vi "Control Valve.vi"(0 "Session Handle in":T2, 5 "Valves":T1=52 items=["GV1"=21, ""=0], 7 "Energize?":bool, 11 "error in (no error)":errorcluster) -> (4 "Session Handle out":T2, 6 "Success?":bool, 15 "error out":errorcluster)   [LabVIEW 2015, in "Gas.lvclass"]
uses:
  Gas.lvclass
  Typedefs/Session Handle.ctl
  Typedefs/Valves.ctl
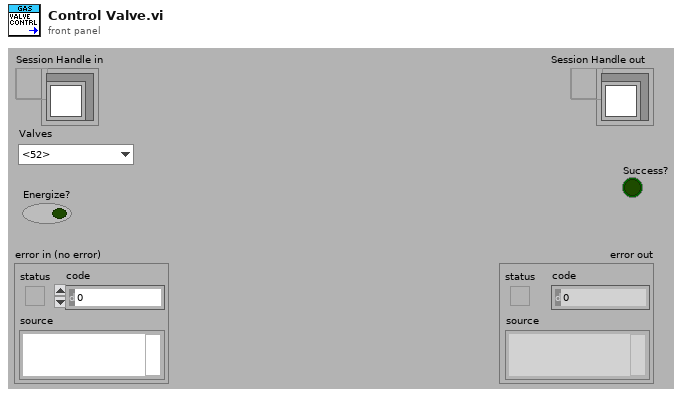
[diagram p1: front panel]
types:
  T1 = typedef "Gas.lvclass/Valves.ctl" = u16
  T2 = typedef "Gas.lvclass/Session Handle.ctl" = refnum<data-value>
  T3 = typedef "XNET Frame CAN.ctl" = cluster{"timestamp":timestamp, "payload":u8[], "identifier":u32, "type":T4, "extended?":bool, "echo?":bool}
  T4 = typedef "XNET Frame Type CAN.ctl" = u8
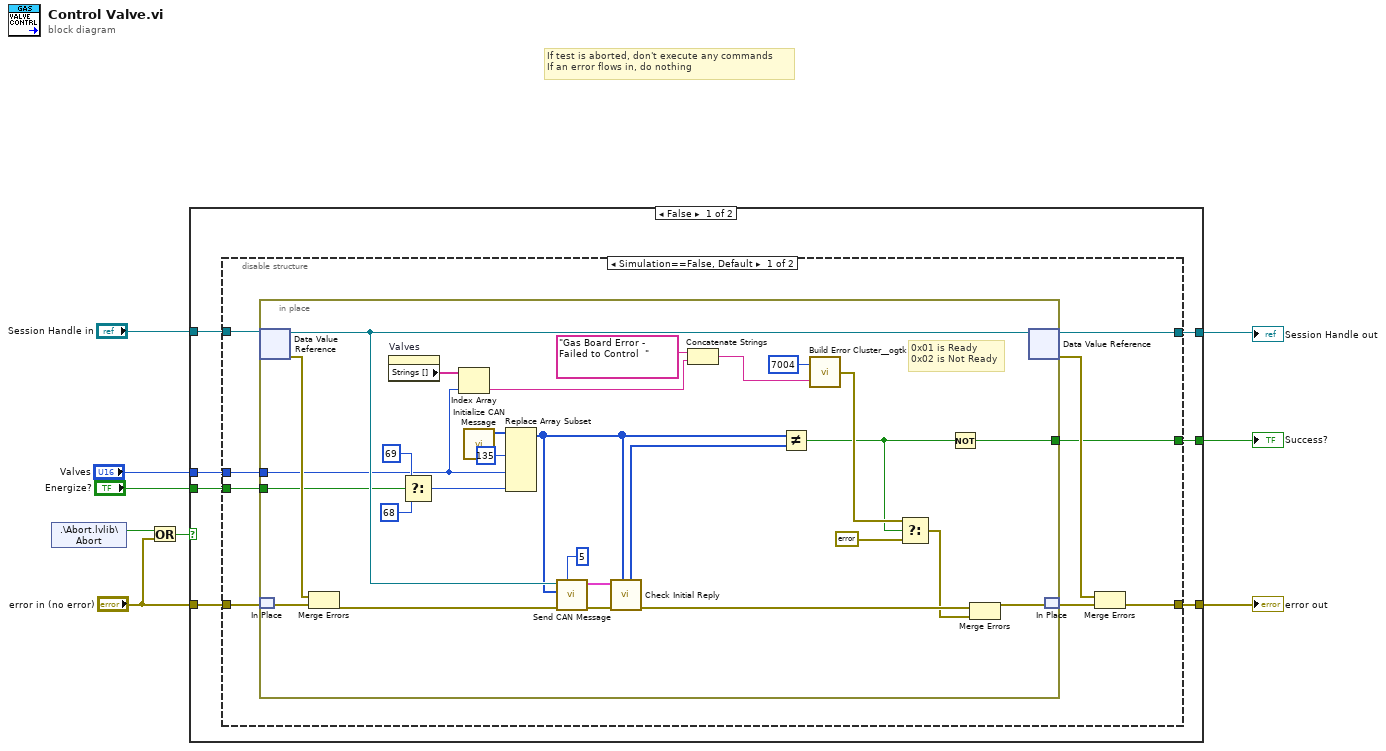
[diagram p0: block diagram]
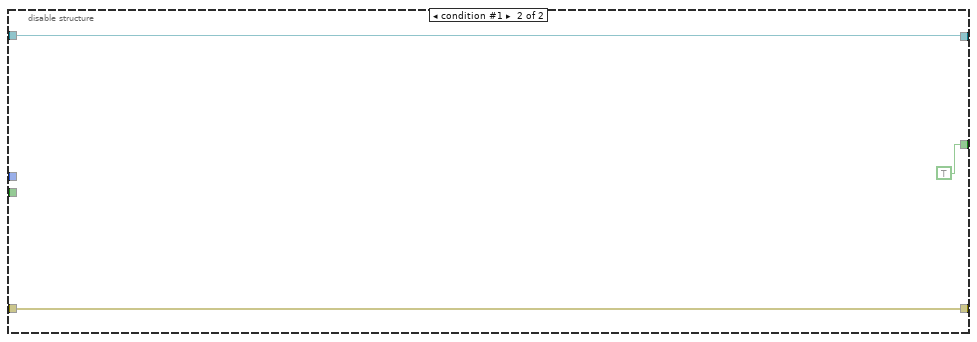
[diagram p2: hidden frame]
diagram:
  # "If test is aborted, don't execute any commands\nIf an error flows in, do nothing"
  n1 = shared-variable ".\\Abort.lvlib\\Abort"() -> (w6:bool)  [unwired: 1 in, 1 out]
  n2 = Or(x=w6, y="error in (no error)") -> (x .or. y?=w4:bool)
  n3 = case shown="False" w4 {
    tunnel: [w16 w58] -> w8
    tunnel: [w15 w57] -> w7
    tunnel: "Session Handle in" -> [w14 w58]
    tunnel: "error in (no error)" -> [w13 w57]
    tunnel: [w12 _] -> w3
    tunnel: "Valves" -> [w11 _]
    tunnel: "Energize?" -> [w10 _]
    frame False {
      n4 = disable-structure shown="Simulation==False, Default" {
        disable-tunnel: [w25 w56] -> w16
        disable-tunnel: [w22 w55] -> w15
        disable-tunnel: w14 -> [w21 w56]
        disable-tunnel: w13 -> [w20 w55]
        disable-tunnel: [w19 TRUE] -> w12
        disable-tunnel: w11 -> [w18 _]
        disable-tunnel: w10 -> [w17 _]
        frame condition #0 (active) {
          n5 = in-place {
            in-place-border: [w40] -> w19
            in-place-border: w18 -> [w32]
            in-place-border: w17 -> [w39]
            # "0x01 is Ready\n0x02 is Not Ready"
            n6 = in-place-dvr #1(w21) -> (w47:refnum<class "Gas.lvclass">, w50:errorcluster)
            n7 = in-place-match #2(w20) -> (w49:errorcluster)
            n8 = Merge Errors(w50, w49) -> (w48:errorcluster)
            n9 = property on="Valves" class="Ring (strict)"() -> ("Strings []"=w33:string[])  [unwired: 2 in, 2 out]
            n10 = Select(t=u8 69 ("new element/subarray"), s=w39, f=u8 68 ("new element/subarray")) -> (s? t:f=w36:u8)
            n11 = Index Array(array=w33, index=w32) -> (element=w30:string)
            n12 = call "Initialize CAN Message.vi"() -> ("Initial Payload"=w51:u8[])  [unwired: 11 in]
            n13 = Replace Array Subset(array=w51, new element #1=u8 135 ("new element/subarray"), new element #2=w32, new element #3=w36) -> (w35:u8[])  [unwired: 3 in]
            n14 = call "Send CAN Message.vi"("Number of Retries"=5, "error in (no error)"=w48, "payload"=w35, "Gas In"=w47) -> ("error out"=w28:errorcluster, "Reply"=w45:T3[])  [unwired: 5 in, 1 out]
            n15 = call "Check Initial Reply.vi"("Write Message"=w35, "error in (no error)"=w28, "Reply"=w45) -> ("error out"=w27:errorcluster, "Whole Payload"=w34:u8[])  [unwired: 5 in, 2 out]
            n16 = Concatenate Strings("Gas Board Error - Failed to Control  " ("string"), w30) -> (w29:string)
            n17 = Not Equal?(x=w35, y=w34) -> (x != y?=w41:bool)
            n18 = call <userlib>:"Build Error Cluster__ogtk.vi"("String to Prepend to source (\"\")"=w29, "code"=7004) -> ("error out"=w43:errorcluster)
            n19 = Select(t=w43, s=w41, f=errorcluster {"status"=FALSE, "code"=0, "source"=""}) -> (s? t:f=w26:errorcluster)
            n20 = Not(x=w41) -> (.not. x?=w40:bool)
            n21 = Merge Errors(w27, w26) -> (w52:errorcluster)
            n22 = in-place-dvr #1(w47) -> (w25:T2, w23:errorcluster)
            n23 = in-place-match #2(w52) -> (w24:errorcluster)
          }
          n24 = Merge Errors(w23, w24) -> (w22:errorcluster)
        }
        frame condition #1 {
        }
      }
    }
    frame True {
    }
  }
  "Session Handle out" <- w8
  "error out" <- w7
  "Success?" <- w3
